vi "variantArrayByRef.vi"(8 "error in (no error)":errorcluster, 10 "Variant":variant, 11 "Array Ref":refnum<vi>) -> (0 "error out":errorcluster, 3 "Array Ref (dup)":refnum<vi>)   [LabVIEW 2015, in "MsgPack.lvlib"]
uses:
  MsgPack.lvlib
  <vilib>/Utility/Data Type/NI_Data Type.lvlib
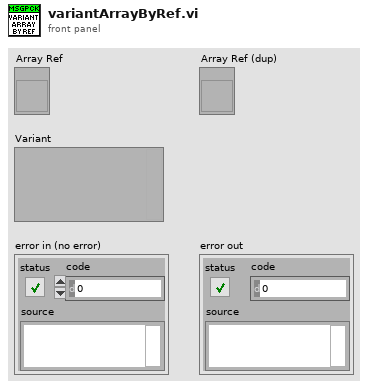
[diagram p1: front panel]
types:
  T1 = typedef "NI_Data Type.lvlib/Data Type.ctl" = enum8{"Invalid Type", "Void", "I8", "I16", "I32", "I64", "U8", "U16", "U32", "U64", "Single Float", "Double Float", "Extended Float", "Single Complex", "Double Complex", "Extended Complex", "Enum U8", "Enum U16", "Enum U32", "Enum U64", "Single Float With Unit", "Double Float With Unit", "Extended Float With Unit", "Single Complex with Unit", "Double Complex with Unit", "Extended Complex with Unit", "Boolean", "String", "Path", "Picture", "Tag", "Array", "Cluster", "Variant", "LV Variant", "Waveform", "Timestamp", "Digital Waveform", "Digital Data", "ExpressData", "Refnum", "External Data", "VI", "Poly VI", "LabVIEW Class Instance", "Fixed Point"}
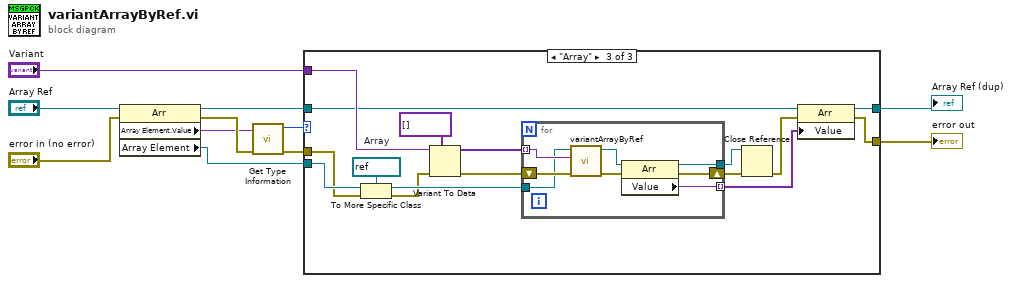
[diagram p0: block diagram]
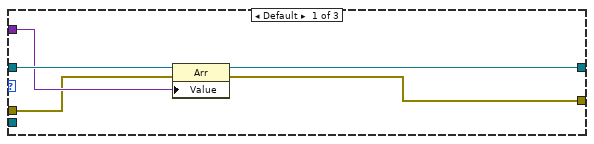
[diagram p2: hidden frame]
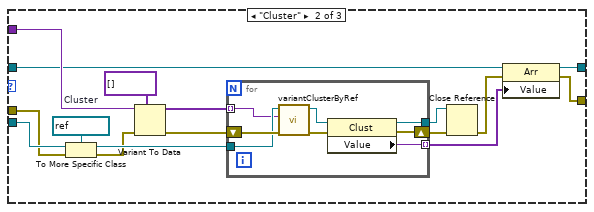
[diagram p3: hidden frame]
diagram:
  n1 = property class="Arr"(reference="Array Ref", error in="error in (no error)") -> (reference out=w6:refnum<vi>, error out=w4:errorcluster, "Array Element.Value"=w3:variant, "Array Element"=w9:refnum<vi>)
  n2 = call <vilib>:"Get Type Information.vi"("error in (no error)"=w4, "Variant"=w3) -> ("error out"=w8:errorcluster, "Type"=w5:T1)  [unwired: 5 in, 3 out]
  n3 = case shown="\"Array\"" w5 {
    tunnel: w6 -> [w16 w23 w47]
    tunnel: "Variant" -> [w15 w32 w56]
    tunnel: w8 -> [w14 w19 w43]
    tunnel: w9 -> [_ w28 w52]
    tunnel: [w13 w20 w44] -> w10
    tunnel: [w12 w17 w41] -> w11
    frame Default {
      n4 = property class="Arr"(reference=w16, error in=w14, "Value"=w15) -> (reference out=w12:refnum<vi>, error out=w13:errorcluster)
    }
    frame "Cluster" {
      w27 = refnum<vi> refnum  # Cluster
      n5 = To More Specific Class(target class=w27, reference=w28, error in=w19) -> (specific class reference=w26:refnum<vi>, error out=w18:errorcluster)
      n6 = Variant To Data(error in=w18, type=variant[] [], Variant=w32) -> (data=w30:variant[], error out=w29:errorcluster)
      n7 = for {
        tunnel: w30 -> [w34] mode=indexing
        shift-right: [w37] -> w24
        shift-left: w29 -> [w40]
        tunnel: w26 -> [w35]
        tunnel: [w38] -> w22 mode=indexing
        tunnel: [w36] -> w25
        n8 = call "variantClusterByRef.vi"("error in (no error)"=w40, "MsgPack Variant"=w34, "Cluster Reference"=w35) -> ("error out"=w39:errorcluster, "Cluster Reference (dup)"=w33:refnum<vi>)  [unwired: 7 in]
        n9 = property class="Clust"(reference=w33, error in=w39) -> (reference out=w36:refnum<vi>, error out=w37:errorcluster, "Value"=w38:variant)
      }
      n10 = Close Reference(reference=w25, error in (no error)=w24) -> (error out=w21:errorcluster)
      n11 = property class="Arr"(reference=w23, error in=w21, "Value"=w22) -> (reference out=w17:refnum<vi>, error out=w20:errorcluster)
    }
    frame "Array" {
      w51 = refnum<vi> refnum  # Array
      n12 = To More Specific Class(target class=w51, reference=w52, error in=w43) -> (specific class reference=w50:refnum<vi>, error out=w42:errorcluster)
      n13 = Variant To Data(error in=w42, type=variant[] [], Variant=w56) -> (data=w54:variant[], error out=w53:errorcluster)
      n14 = for {
        tunnel: w54 -> [w60] mode=indexing
        shift-right: [w63] -> w48
        shift-left: w53 -> [w61]
        tunnel: w50 -> [w59]
        tunnel: [w64] -> w46 mode=indexing
        tunnel: [w62] -> w49
        n15 = call "variantArrayByRef.vi"("error in (no error)"=w61, "Variant"=w60, "Array Ref"=w59) -> ("error out"=w57:errorcluster, "Array Ref (dup)"=w58:refnum<vi>)  [unwired: 7 in]
        n16 = property class="Arr"(reference=w58, error in=w57) -> (reference out=w62:refnum<vi>, error out=w63:errorcluster, "Value"=w64:variant)
      }
      n17 = Close Reference(reference=w49, error in (no error)=w48) -> (error out=w45:errorcluster)
      n18 = property class="Arr"(reference=w47, error in=w45, "Value"=w46) -> (reference out=w41:refnum<vi>, error out=w44:errorcluster)
    }
  }
  "Array Ref (dup)" <- w11
  "error out" <- w10
